vi "A 侧面 处理函数CCDA.vi"(8 "error in (no error)":errorcluster caption="错误输入（无错误）", 10 "Image Name":string="I1", 11 "ParamsUI":T2={"IsNorImage"=TRUE, "Exposure Values"=100289, "ImagePath"=path "C:/Users/hedongpo/Desktop/514-hdp/Alignment Assemble System/Test Picture/B/3.bmp"} caption="参数界面" {"Exposure Values" scale=0.0..200000.0}) -> (0 "error out":errorcluster caption="错误输出", 2 "Session Out":T1, 3 "Image out":T3(plugin-control), 4 "数值":dbl)   [LabVIEW 2017]
uses:
  <vilib>/userdefined/High Color/IMAQdx.ctl
  <vilib>/vision/driver/IMAQdx.llb/IMAQdx Buffer Number Mode.ctl
  Global System.vi
  <resource>/objmgr/imaqdx.rc
  <vilib>/vision/driver/NI_Vision_Acquisition_Software.lvlib
  <vilib>/vision/NI_Vision_Development_Module.lvlib
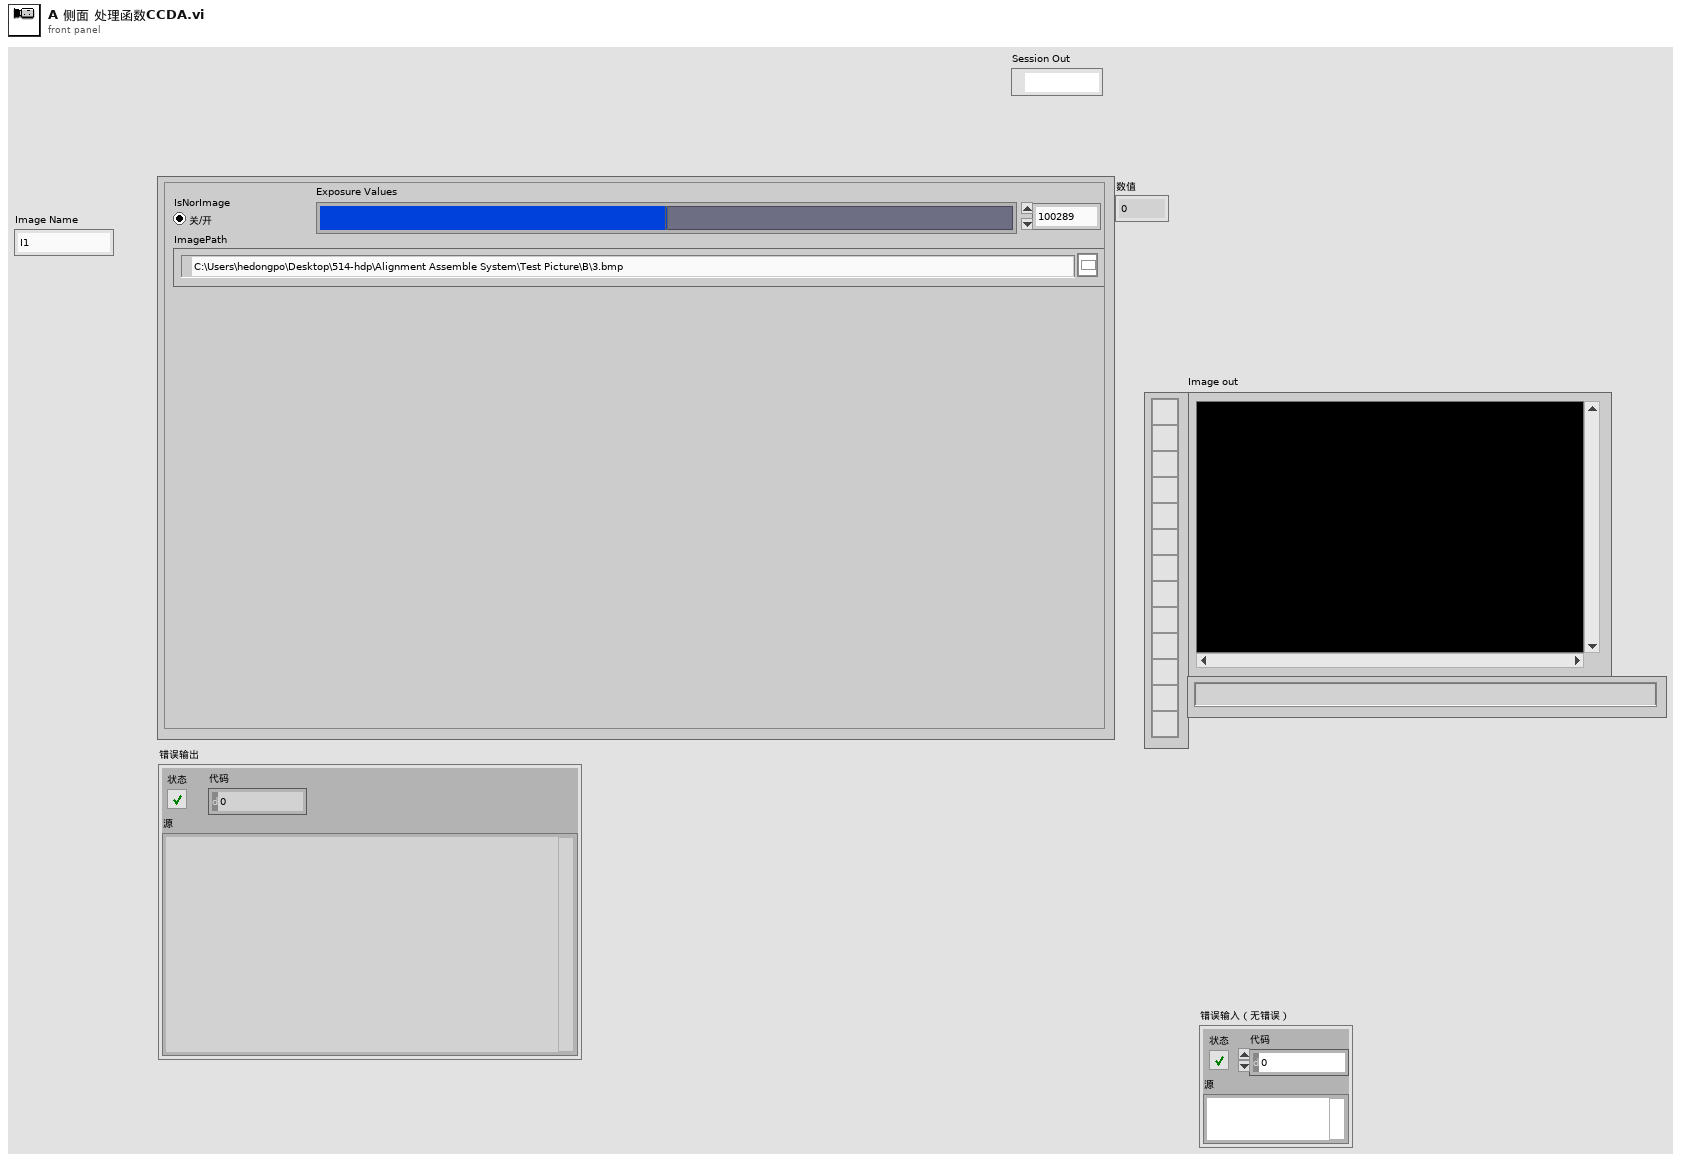
[diagram p1: front panel]
types:
  T1 = typedef "IMAQdx.ctl" = refnum<k21>
  T2 = cluster{"IsNorImage":bool, "Exposure Values":i64, "ImagePath":path}
  T3 = typedef "IMAQ Image.ctl" = refnum<image>
  T4 = typedef "Image Type" = u32
  T5 = cluster{"IsNorImage":bool, "Exposure Values":u32, "ImagePath":path}
  T6 = typedef "NI_Vision_Acquisition_Software.lvlib/IMAQdx Buffer Number Mode.ctl" = enum32{"Next", "Last", "Buffer Number", "Every", "Last New"}
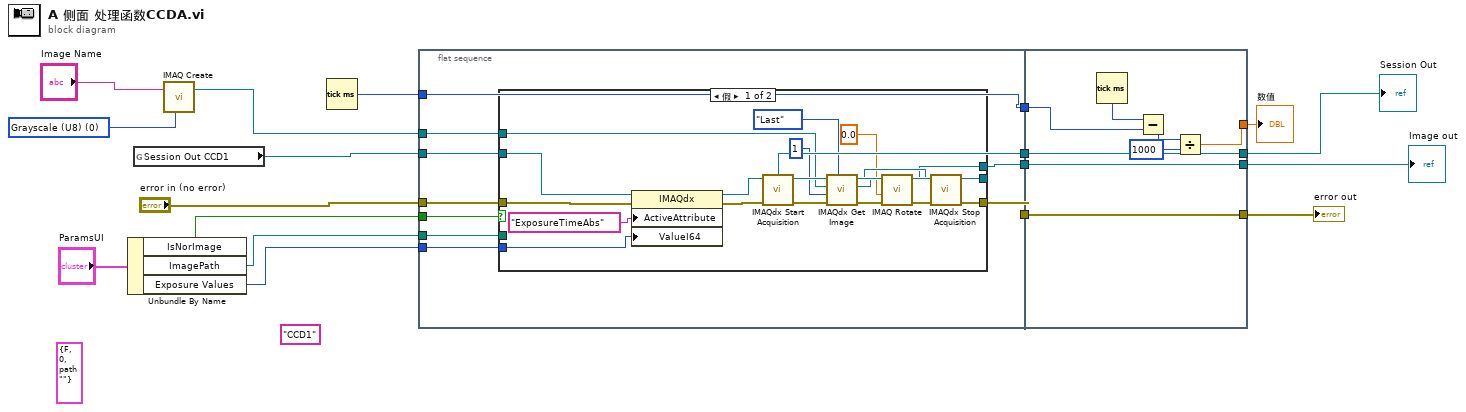
[diagram p0: block diagram]
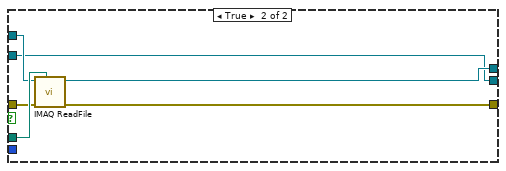
[diagram p2: hidden frame]
diagram:
  (unwired) "CCD1"
  w13 = T4 0 items=["Grayscale (U8)", "Grayscale (I16)", "Grayscale (SGL)", "Complex (CSG)", "RGB (U32)", "HSL (U32)", "RGB (U64)", "Grayscale (U16)"] ("Image Type")
  (unwired) T5 {"IsNorImage"=FALSE, "Exposure Values"=0, "ImagePath"=path ""} ("ParamsUI")
  n1 = Unbundle By Name("ParamsUI") -> ("IsNorImage"=w1:bool, "ImagePath"=w2:path, "Exposure Values"=w18:i64)
  n2 = global read "Global System.vi" "Session Out CCD1"() -> (w10:T1)
  n3 = call "IMAQ Create"("Image Name"="Image Name", "Image Type"=w13) -> ("New Image"=w16:T3)  [unwired: 3 in, 1 out]
  n4 = Tick Count (ms)() -> (millisecond timer value=w8:u32)
  n5 = flat-sequence {
    tunnel: w1 -> [w28]
    tunnel: w2 -> [w27]
    tunnel: w18 -> [w26]
    tunnel: w16 -> [w25]
    tunnel: "error in (no error)" -> [w24]
    tunnel: w10 -> [w21]
    tunnel: w8 -> [w19]
    tunnel: [w23] -> w7
    tunnel: [w22] -> w6
    tunnel: [w20] -> w5
    tunnel: [w19] -> w4
    tunnel: [w59] -> w9
    tunnel: [w60] -> w11
    tunnel: [w61] -> w14
    tunnel: w7 -> [w61]
    tunnel: w6 -> [w60]
    tunnel: w5 -> [w59]
    tunnel: w4 -> [w57]
    tunnel: [w54] -> w3
    frame #0 {
      n6 = case shown="假" w28 {
        tunnel: w27 -> [_ w53]
        tunnel: [w37 w52] -> w22
        tunnel: w26 -> [w32 _]
        tunnel: w21 -> [w34 w48]
        tunnel: w25 -> [w38 w51]
        tunnel: w24 -> [w33 w50]
        tunnel: [w35 w49] -> w23
        tunnel: [w36 w48] -> w20
        frame False {
          n7 = property class="IMAQdx"(reference=w34, error in=w33, "ActiveAttribute"="ExposureTimeAbs", "ValueI64"=w32) -> (reference out=w31:T1, error out=w30:errorcluster)
          n8 = call <vilib>:"IMAQdx Start Acquisition.vi"("error in"=w30, "Session In"=w31) -> ("error out"=w46:errorcluster, "Session Out"=w47:T1)  [unwired: 8 in]
          n9 = call <vilib>:"IMAQdx Get Image.vi"("Buffer Number Mode (Next)"=IMAQdx_Buffer_Number_Mode."Last", "error in"=w46, "Buffer Number In"=u32 1, "Image In"=w38, "Session In"=w47) -> ("error out"=w41:errorcluster, "Image Out"=w42:T3, "Session Out"=w43:T1)  [unwired: 3 in, 1 out]
          n10 = call "IMAQ Rotate"("error in (no error)"=w41, "Angle (degrees)"=sgl 0.0, "Image Src"=w42) -> ("error out"=w40:errorcluster, "Image Dst Out"=w37:T3)  [unwired: 7 in]
          n11 = call <vilib>:"IMAQdx Stop Acquisition.vi"("error in"=w40, "Session In"=w43) -> ("error out"=w35:errorcluster, "Session Out"=w36:T1)  [unwired: 8 in]
        }
        frame True {
          n12 = call "IMAQ ReadFile"("File Path"=w53, "error in (no error)"=w50, "Image"=w51) -> ("error out"=w49:errorcluster, "Image Out"=w52:T3)  [unwired: 4 in, 3 out]
        }
      }
    }
    frame #1 {
      n13 = Tick Count (ms)() -> (millisecond timer value=w58:u32)
      n14 = Subtract(x=w58, y=w57) -> (x-y=w56:u32)
      n15 = Divide(x=w56, y=u32 1000) -> (x/y=w54:dbl)
    }
  }
  "Image out" <- w11
  "error out" <- w14
  "Session Out" <- w9
  "数值" <- w3
